vi "Communication To Controller.vi"(8 "error in":errorcluster, 10 "Data":variant, 11 "Command":string) -> (0 "error out":errorcluster)   [LabVIEW 2020, in "DisplayConsole.lvlib"]
doc: "Uses the communication Manager FGV, to send a message to a module using one of its queue references"
uses:
  DisplayConsole.lvlib
  Controls/Module QMsg.ctl
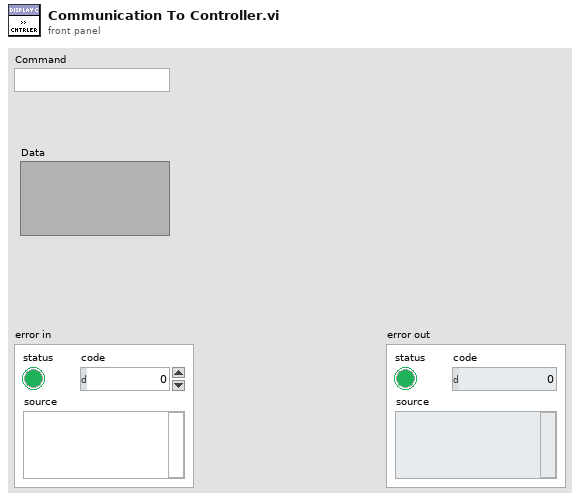
[diagram p1: front panel]
types:
  T1 = typedef "DisplayConsole.lvlib/Module QMsg.ctl" = cluster{"Command":string, "Data":variant}
  T2 = typedef "DisplayConsole.lvlib/Module Messaging Structures.ctl" = cluster{">>EventHandlers":refnum<user-event>, ">>ErrorQ":refnum<queue>}
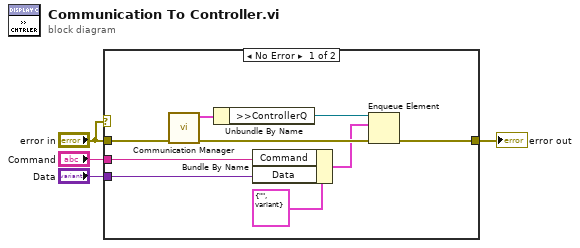
[diagram p0: block diagram]
diagram:
  n1 = case shown="No Error" "error in" {
    tunnel: "error in" -> [w9 w14]
    tunnel: [w11 w14] -> w3
    tunnel: "Data" -> [w6 _]
    tunnel: "Command" -> [w5 _]
    frame No Error {
      n2 = call "Communication Manager.vi"("error in"=w9) -> ("error out"=w10:errorcluster, "Messaging Structures"=w13:T2)  [unwired: 9 in]
      n3 = Unbundle By Name(w13) -> (">>ControllerQ"=w12:refnum<queue>)
      n4 = Bundle By Name(cluster=T1 {"Command"="", "Data"=variant} ("element"), "Command"=w5, "Data"=w6) -> (w7:T1)
      n5 = Enqueue Element(queue=w12, element=w7, error in (no error)=w10) -> (error out=w11:errorcluster)  [unwired: 1 in, 2 out]
    }
    frame Error {
    }
  }
  "error out" <- w3
